vi "Read-Write_Check_Pos.vi"(1 "Position input":sgl[](array[numeric]), 2 "Mode":enum16{"Read", "Write"}(ring), 3 "Traverse Name":string="EnFlo Tunnel") -> (0 "Position Output":sgl[](array[numeric]))   [LabVIEW 2014]
uses:
  Globals/Constants_global.vi
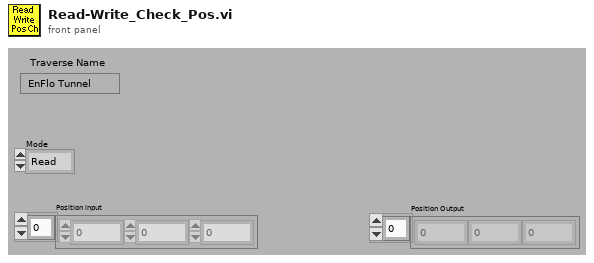
[diagram p1: front panel]
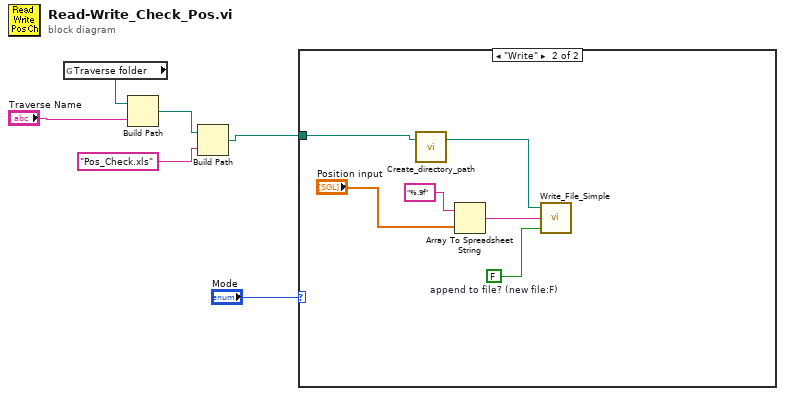
[diagram p0: block diagram]
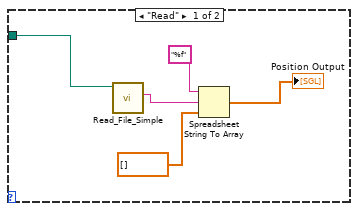
[diagram p2: hidden frame]
diagram:
  n1 = global read "Constants_global.vi" "Traverse folder"() -> (w6:path)
  n2 = Build Path(base path=w6, name or relative path="Traverse Name") -> (appended path=w5:path)
  n3 = Build Path(base path=w5, name or relative path="Pos_Check.xls" ("string")) -> (appended path=w4:path)
  n4 = case shown="\"Write\"" "Mode" {
    tunnel: w4 -> [w11 w15]
    frame "Read" {
      n5 = call "Read_File_Simple.vi"("Filename"=w11) -> ("string"=w10:string)  [unwired: 2 in, 7 out]
      n6 = Spreadsheet String To Array(format string="%f", spreadsheet string=w10, array type (2D Dbl)=sgl[] []) -> (array=→"Position Output":sgl[])  [unwired: 1 out]
    }
    frame "Write" {
      w17 = FALSE  # append to file? (new file:F)
      n7 = call "Create_directory_path.vi"("Path name"=w15) -> ("Path name Out"=w14:path)  [unwired: 1 in, 1 out]
      n8 = Array To Spreadsheet String(array="Position input", 3:"%.9f" ("format string")) -> (spreadsheet string=w16:string)  [unwired: 1 out]
      n9 = call "Write_File_Simple.vi"("append to file? (new file:F)"=w17, "character string"=w16, "file path"=w14) -> ()  [unwired: 2 out]
    }
  }
